vi "Option Parser.vi"(0 "Yokogawa WT2X0 in":refnum<class "Yokogawa WT2X0.lvclass">, 1 "ID":string, 2 "THD?":bool, 3 "Number of Cards":dbl, 4 "ID cluster.Model":string, 5 "error in (no error)":errorcluster, 7 "Option":string) -> (14 "Yokogawa WT2X0 out":refnum<class "Yokogawa WT2X0.lvclass">, 19 "error out":errorcluster)   [LabVIEW 2016, in "Generic Power Analyzer.lvlib" / "Yokogawa WT2X0.lvlib" / "Yokogawa WT2X0.lvclass"]
uses:
  Yokogawa WT2X0.lvclass
panel:
  out "f":dbl
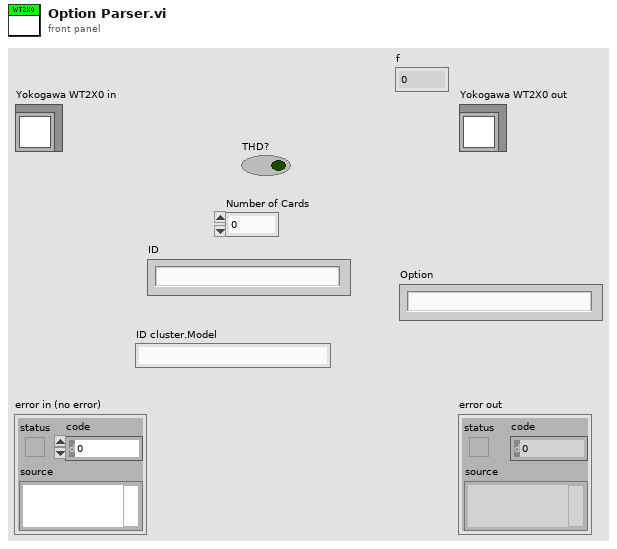
[diagram p1: front panel]
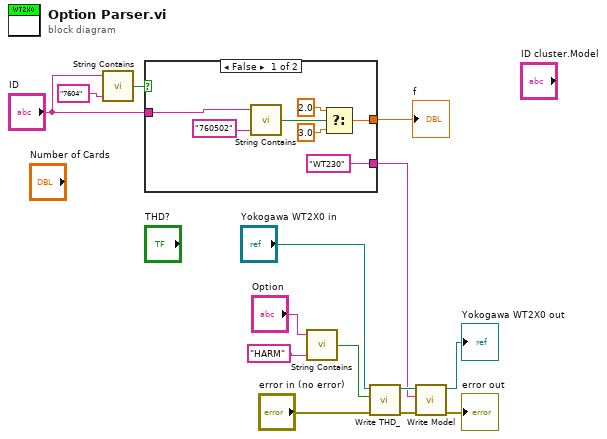
[diagram p0: block diagram]
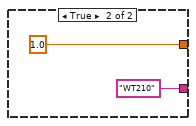
[diagram p2: hidden frame]
diagram:
  n1 = call "String Contains.vi"("Regular expression"="7604" ("Expression to evaluate"), "Input String"="ID") -> ("Found?"=w13:bool)  [unwired: 2 in, 1 out]
  n2 = case shown="False" w13 {
    tunnel: [w16 1.0] -> w11
    tunnel: "ID" -> [w21 _]
    tunnel: ["WT230" "WT210"] -> w3
    frame False {
      n3 = call "String Contains.vi"("Regular expression"="760502" ("Expression to evaluate"), "Input String"=w21) -> ("Found?"=w19:bool)  [unwired: 2 in, 1 out]
      n4 = Select(t=2.0, s=w19, f=3.0) -> (s? t:f=w16:dbl)
    }
    frame True {
    }
  }
  "f" <- w11
  n5 = call "String Contains.vi"("Regular expression"="HARM" ("Expression to evaluate"), "Input String"="Option") -> ("Found?"=w7:bool)  [unwired: 2 in, 1 out]
  n6 = call-dynamic "Write THD_.vi"("error in (no error)"="error in (no error)", "THD?"=w7, "Generic Power Analyzer in"="Yokogawa WT2X0 in") -> ("error out"=w2:errorcluster, "Generic Power Analyzer out"=w5:refnum<class "Yokogawa WT2X0.lvclass">)  [unwired: 7 in]
  n7 = call-dynamic "Write Model.vi"("error in (no error)"=w2, "Model"=w3, "Generic Device in"=w5) -> ("error out"=→"error out":errorcluster, "Generic Device out"=→"Yokogawa WT2X0 out":refnum<class "Yokogawa WT2X0.lvclass">)  [unwired: 7 in]
